vi "open.vi"(1 "地址":string) -> (0 "连接ID":refnum<k5>)   [LabVIEW 2017]
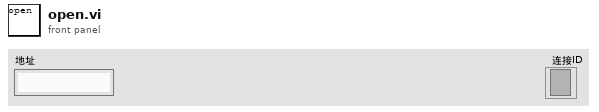
[diagram p1: front panel]
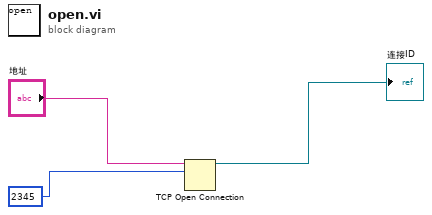
[diagram p0: block diagram]
diagram:
  n1 = TCP Open Connection(address="地址", remote port or service name=u16 2345 ("远程端口或服务名称")) -> (connection ID=→"连接ID":refnum<k5>)  [unwired: 3 in, 1 out]
